vi "Micron Optics sm130 Convert Sensor Wavelength.vi"() -> ()   [LabVIEW 2015]
doc: "Demonstrates converting the wavelength of one strain sensor and one temperature compensation sensor to Strain Measurement.\n\n<b>Note:</b>\nThis example is made for the instrument without channel multiplexer. Modifications will have to be made for instruments with channel multiplexer."
uses:
  Micron Optics sm130.lvlib
panel:
  in  "Sample Rate (1000 Hz)":i32=1000
  in  "Null":bool
  out "Strain Chart":dbl(graph)
  in  "Strain Nominal Wavelength (0 nm)":dbl format="%#_10g"
  in  "Temperature Nominal Wavelength (0 nm)":dbl format="%#_10g"
  in  "Gage Constant 2 (0.7)":dbl=0.7
  in  "Gage Constant 1 (6.156)":dbl=6.156
  in  "Gage Factor (0.89)":dbl=0.89
  in  "CTE of Test Specimen (0)":dbl
  in  "Stop":bool
  in  "Channel (1: Channel 1)":i32(ring)=1 items=["Channel 1"=1, "Channel 2"=2, "Channel 3"=3, "Channel 4"=4]
  in  "VISA resource name":refnum<visa-resource-name>
  # "(c) 2009 - 2012 National Instruments.  ALL RIGHTS RESERVED."
  # "Sensor Setup"
  # "• This example demonstrates converting the wavelength of one strain sensor and one temperature compensation sensor to Strain Measurement.\n• Before running this example, enter the sensor setup constants obtained from the Sensor Information Sheet. \n• Modification to this example is needed to display strain measurement for multiple strain sensors."
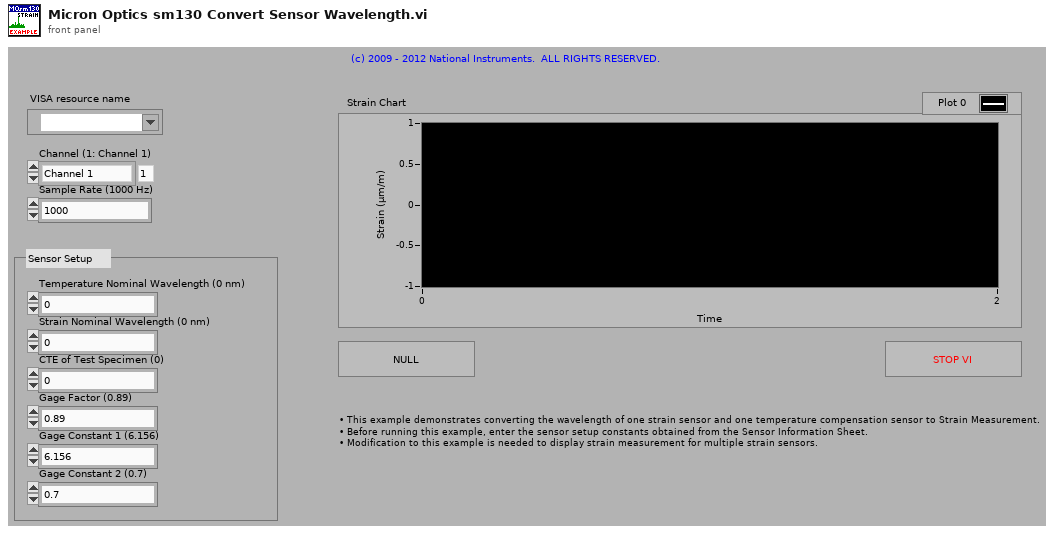
[diagram p1: front panel]
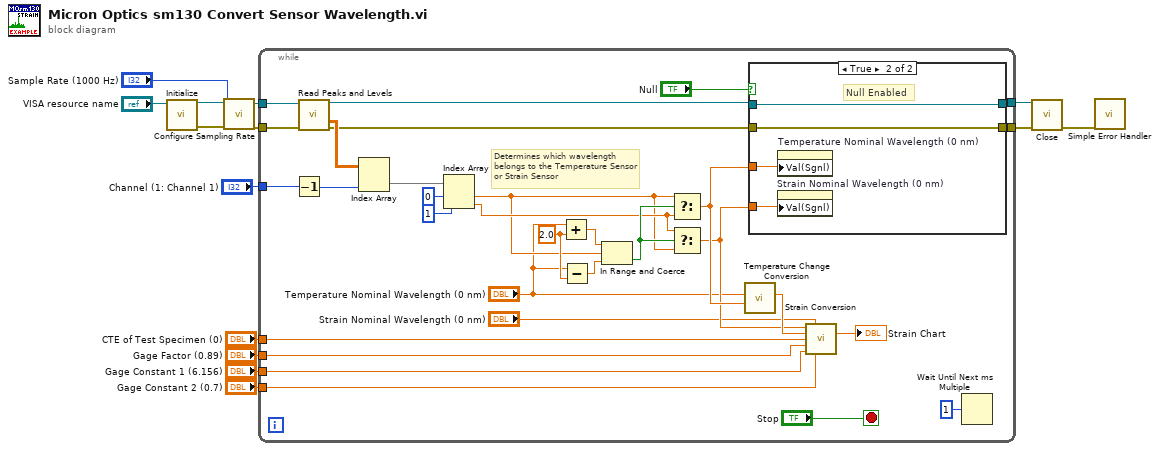
[diagram p0: block diagram]
diagram:
  n1 = call "Initialize.vi"("VISA resource name"="VISA resource name") -> ("error out"=w11:errorcluster, "VISA resource name out"=w10:refnum<visa-resource-name>)  [unwired: 9 in]
  n2 = call "Configure Sampling Rate.vi"("error in (no error)"=w11, "Sample Rate (1000 Hz)"="Sample Rate (1000 Hz)", "VISA resource name"=w10) -> ("error out"=w12:errorcluster, "VISA resource name out"=w13:refnum<visa-resource-name>)  [unwired: 7 in]
  n3 = while {
    tunnel: w13 -> [w45]
    tunnel: w12 -> [w44]
    tunnel: [w23] -> w3
    tunnel: [w21] -> w2
    tunnel: "Channel (1: Channel 1)" -> [w30]
    tunnel: "CTE of Test Specimen (0)" -> [w29]
    tunnel: "Gage Factor (0.89)" -> [w28]
    tunnel: "Gage Constant 1 (6.156)" -> [w27]
    tunnel: "Gage Constant 2 (0.7)" -> [w26]
    stop <- "Stop" stop-if-true
    w35 = 2.0 ("y")
    # "Determines which wavelength belongs to the Temperature Sensor or Strain Sensor"
    n4 = Decrement(x=w30) -> (x-1=w15:i32)
    n5 = call "Read Peaks and Levels.vi"("VISA resource name"=w45, "error in (no error)"=w44) -> ("VISA resource name out"=w24:refnum<visa-resource-name>, "Peak Wavelengths (nm)"=w41:dbl[][], "error out"=w22:errorcluster)  [unwired: 5 in, 6 out]
    n6 = Index Array(array=w41, index (col)=w15) -> (element=w40:dbl[])  [unwired: 1 in]
    n7 = Index Array(array=w40, index #1=0 ("index"), index #2=1 ("index")) -> (element #1=w32:dbl, element #2=w33:dbl)
    n8 = Add(x="Temperature Nominal Wavelength (0 nm)", y=w35) -> (x+y=w37:dbl)
    n9 = Subtract(x="Temperature Nominal Wavelength (0 nm)", y=w35) -> (x-y=w36:dbl)
    n10 = In Range and Coerce(upper limit=w37, x=w32, lower limit=w36) -> (In Range?=w34:bool)  [unwired: 1 out]
    n11 = Select(t=w32, s=w34, f=w33) -> (s? t:f=w20:dbl)
    n12 = Select(t=w33, s=w34, f=w32) -> (s? t:f=w19:dbl)
    n13 = call "Temperature Change Conversion.vi"("Current Wavelength (0 nm)"=w20, "Nominal Wavelength (0 nm)"="Temperature Nominal Wavelength (0 nm)") -> ("Temperature Change (°C)"=w42:dbl)  [unwired: 9 in]
    n14 = case shown="True" "Null" {
      tunnel: w24 -> [w47 w51]
      tunnel: [w47 w51] -> w23
      tunnel: w22 -> [w46 w49]
      tunnel: [w46 w49] -> w21
      tunnel: w20 -> [_ w50]
      tunnel: w19 -> [_ w48]
      frame False {
        # "No Nulling"
      }
      frame True {
        # "Null Enabled"
        n15 = property on="Temperature Nominal Wavelength (0 nm)" class="DigNum (strict)"("Val(Sgnl)"=w50) -> ()  [unwired: 2 in, 2 out]
        n16 = property on="Strain Nominal Wavelength (0 nm)" class="DigNum (strict)"("Val(Sgnl)"=w48) -> ()  [unwired: 2 in, 2 out]
      }
    }
    n17 = call "Strain Conversion.vi"("Current Wavelength (0 nm)"=w19, "Nominal Wavelength (0 nm)"="Strain Nominal Wavelength (0 nm)", "Temperature Change (°C)"=w42, "CTE of Test Specimen (0)"=w29, "Gage Factor (0.89)"=w28, "Gage Constant 1 (6.156)"=w27, "Gage Constant 2 (0.7)"=w26) -> ("Strain (µm/m)"=→"Strain Chart":dbl)  [unwired: 8 in]
    n18 = Wait Until Next ms Multiple(millisecond multiple=u32 1) -> ()  [unwired: 1 out]
  }
  n19 = call "Close.vi"("error in (no error)"=w2, "VISA resource name"=w3) -> ("error out"=w1:errorcluster)  [unwired: 9 in]
  n20 = call <vilib>:"Simple Error Handler.vi"("error in (no error)"=w1) -> ()  [unwired: 4 in, 5 out]
